vi "sv_UFF58 Check Data Valid (Generic).vi"(5 "ordinate values (Y Real)":dbl[](array[numeric]), 7 "ordinate values (Y Im)":dbl[](array[numeric]), 11 "error in (no error)":errorcluster) -> (3 "real or complex data?":enum16{"Real data", "Complex data"}(ring), 6 "dup ordinate values (Y Real)":dbl[](array[numeric]), 8 "dup ordinate values (Y Im)":dbl[](array[numeric]), 15 "error out":errorcluster)   [LabVIEW 2017, in "SoundVib_UFF58.lvlib"]
uses:
  <vilib>/addons/Sound and Vibration/svt_UFF58/SoundVib_UFF58.lvlib
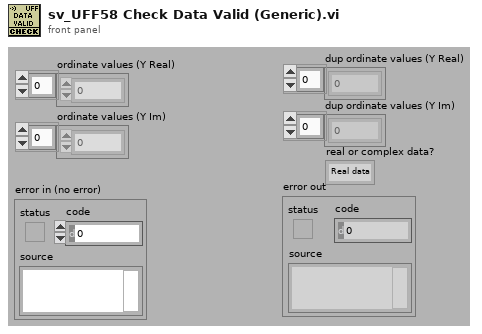
[diagram p1: front panel]
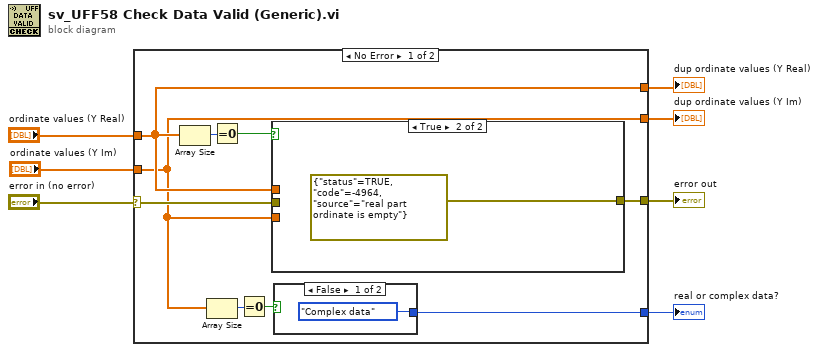
[diagram p0: block diagram]
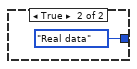
[diagram p2: hidden frame]
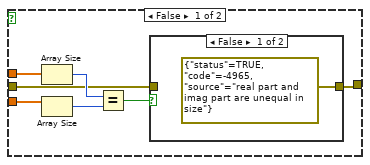
[diagram p3: hidden frame]
diagram:
  n1 = case shown="No Error" "error in (no error)" {
    selector: "error in (no error)" -> [w15 w31]
    tunnel: "ordinate values (Y Real)" -> [w13 w30]
    tunnel: [w16 w31] -> w7
    tunnel: [w13 w30] -> w3
    tunnel: "ordinate values (Y Im)" -> [w10 w29]
    tunnel: [w10 w29] -> w2
    tunnel: [w8 _] -> w1
    frame No Error {
      n2 = Array Size(array=w13) -> (size(s)=w14:i32)
      n3 = Array Size(array=w10) -> (size(s)=w11:i32)
      n4 = Equal To 0?(x=w14) -> (x = 0?=w12:bool)
      n5 = Equal To 0?(x=w11) -> (x = 0?=w9:bool)
      n6 = case shown="True" w12 {
        tunnel: w15 -> [w21 _]
        tunnel: [w19 errorcluster {"status"=TRUE, "code"=-4964, "source"="real part ordinate is empty"} ("error IO")] -> w16
        tunnel: w13 -> [w25 _]
        tunnel: w10 -> [w24 _]
        frame False {
          n7 = Array Size(array=w25) -> (size(s)=w23:i32)
          n8 = Array Size(array=w24) -> (size(s)=w22:i32)
          n9 = Equal?(x=w23, y=w22) -> (x = y?=w20:bool)
          n10 = case shown="False" w20 {
            tunnel: w21 -> [_ w27]
            tunnel: [errorcluster {"status"=TRUE, "code"=-4965, "source"="real part and imag part are unequal in size"} ("error IO") w27] -> w19
            frame False {
            }
            frame True {
              # "real and imag sizes are equal"
            }
          }
        }
        frame True {
        }
      }
      n11 = case shown="False" w9 {
        tunnel: [enum16{"Real data", "Complex data"}."Complex data" ("real or complex data?") enum16{"Real data", "Complex data"}."Real data" ("real or complex data?")] -> w8
        frame False {
        }
        frame True {
        }
      }
    }
    frame Error {
    }
  }
  "error out" <- w7
  "dup ordinate values (Y Real)" <- w3
  "dup ordinate values (Y Im)" <- w2
  "real or complex data?" <- w1
